vi "Set XY Accleration.vi"(8 "error in (no error)":errorcluster, 10 "mm/s":dbl=200.0 format="%#_13g", 11 "A3200 in":refnum<class "A3200.lvclass">) -> (0 "error out":errorcluster, 3 "A3200 out":refnum<class "A3200.lvclass">)   [LabVIEW 2016, in "A3200.lvclass"]
uses:
  A3200.lvclass
  A3200.lvclass/A3200.ctl
  Drivers/Aerotech A3200/Aerotech VIs.lvlib
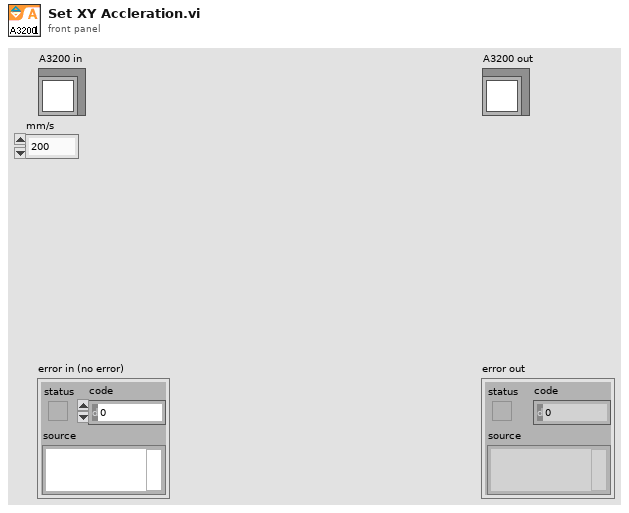
[diagram p1: front panel]
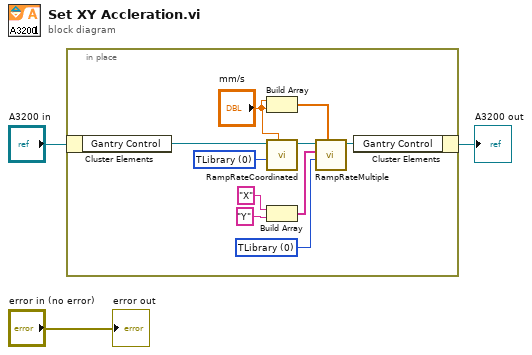
[diagram p0: block diagram]
diagram:
  n1 = in-place {
    w11 = 0 items=["TLibrary", "T01", "T02", "T03", "T04", "T05", "T06", "T07", "T08", "T09", "T10", "T11", "T12", "T13", "T14", "T15", "T16", "T17", "T18", "T19", "T20", "T21", "T22", "T23", "T24", "T25", "T26", "T27", "T28", "T29", "T30", "T31"] ("task id")
    w12 = 0 items=["TLibrary", "T01", "T02", "T03", "T04", "T05", "T06", "T07", "T08", "T09", "T10", "T11", "T12", "T13", "T14", "T15", "T16", "T17", "T18", "T19", "T20", "T21", "T22", "T23", "T24", "T25", "T26", "T27", "T28", "T29", "T30", "T31"] ("taskId")
    n2 = in-place-cluster #1("A3200 in") -> ("Gantry Control"=w6:refnum<k24>)
    n3 = Build Array("mm/s", "mm/s") -> (w13:dbl[])
    n4 = call "RampRateCoordinated.vi"("ramp rate"="mm/s", "taskId"=w12, "controller in"=w6) -> ("controller out"=w10:refnum<k24>)  [unwired: 7 in, 1 out]
    n5 = Build Array("X", "Y") -> (w7:string[])
    n6 = call "RampRateMultiple.vi"("ramp rates"=w13, "task id"=w11, "axis names"=w7, "controller in"=w10) -> ("controller out"=w5:refnum<k24>)  [unwired: 6 in, 1 out]
    n7 = in-place-cluster #1("Gantry Control"=w5) -> (→"A3200 out":refnum<class "A3200.lvclass">)
  }
  "error out" <- "error in (no error)"
